vi "json vaj rxy enable.vi"(11 "<JSON> in":string) -> (0 "VAJ":dbl[](array[numeric]), 1 "enable <R,X,Y>":bool[](array[boolean]), 3 "<JSON> out":string, 4 "enable\nnowcoordinate":bool)   [LabVIEW 2019]
uses:
  <vilib>/JDP Science/JSONtext/JSONtext.lvlib
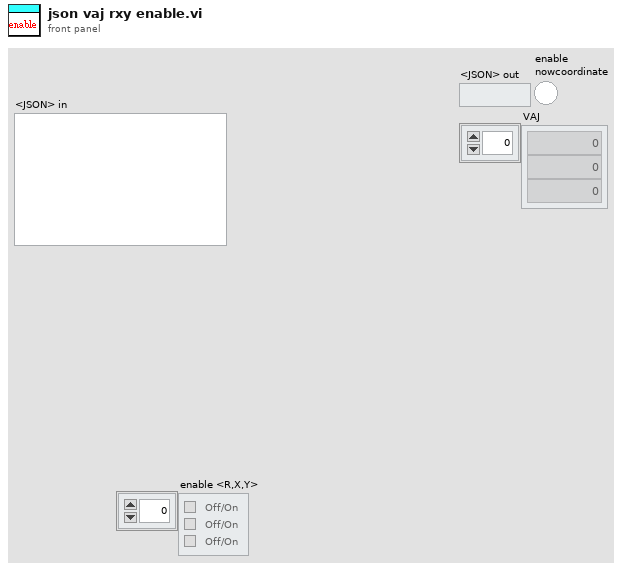
[diagram p1: front panel]
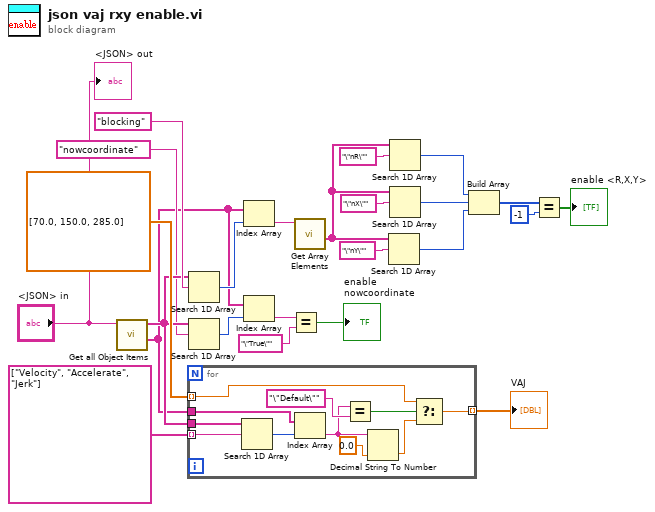
[diagram p0: block diagram]
diagram:
  n1 = call <vilib>:"Get all Object Items.vi"("JSON"="<JSON> in") -> ("<JSON>"=w4:string[], "Item Names"=w6:string[])  [unwired: 7 in, 2 out]
  n2 = for {
    tunnel: string[] ["Velocity", "Accelerate", "Jerk"] ("element") -> [w34] mode=indexing
    tunnel: w6 -> [w33]
    tunnel: w4 -> [w32]
    tunnel: dbl[] [70.0, 150.0, 285.0] -> [w29] mode=indexing
    tunnel: [w25] -> w8 mode=indexing
    n3 = Search 1D Array(1D array=w33, element=w34) -> (index of element=w35:i32)  [unwired: 1 in]
    n4 = Index Array(array=w32, index=w35) -> (element=w28:string)
    n5 = Equal?(x=w28, y="\"Default\"") -> (x = y?=w30:bool)
    n6 = Decimal String To Number(string=w28, default (0L)=0.0 ("default (0 I32)")) -> (number=w26:dbl)  [unwired: 1 in, 1 out]
    n7 = Select(t=w29, s=w30, f=w26) -> (s? t:f=w25:dbl)
  }
  "VAJ" <- w8
  n8 = Search 1D Array(1D array=w6, element="blocking") -> (index of element=w13:i32)  [unwired: 1 in]
  n9 = Search 1D Array(1D array=w6, element="nowcoordinate") -> (index of element=w7:i32)  [unwired: 1 in]
  n10 = Index Array(array=w4, index=w13) -> (element=w14:string)
  n11 = Index Array(array=w4, index=w7) -> (element=w3:string)
  n12 = Equal?(x=w3, y="\"True\"") -> (x = y?=→"enable\nnowcoordinate":bool)
  n13 = call <vilib>:"Get Array Elements.vi"("JSON"=w14) -> ("<JSON>"=w15:string[])  [unwired: 8 in, 2 out]
  n14 = Search 1D Array(1D array=w15, element="\"nY\"") -> (index of element=w21:i32)  [unwired: 1 in]
  n15 = Search 1D Array(1D array=w15, element="\"nR\"") -> (index of element=w19:i32)  [unwired: 1 in]
  n16 = Search 1D Array(1D array=w15, element="\"nX\"") -> (index of element=w20:i32)  [unwired: 1 in]
  n17 = Build Array(w19, w20, w21) -> (w22:i32[])
  n18 = Equal?(x=w22, y=-1) -> (x = y?=→"enable <R,X,Y>":bool[])
  "<JSON> out" <- "<JSON> in"
